vi "Run Filter.vi"(8 "error in (no error)":errorcluster, 10 "fpga resources in":T1[](array[typedef]), 11 "OR Filter in":refnum<class "OR Filter.lvclass">) -> (0 "error out":errorcluster, 2 "fpga resources in":T1[](array[typedef]))   [LabVIEW 2016, in "OR Filter.lvclass"]
uses:
  OR Filter.lvclass
  FPGA-Addon/Source/System Explorer/SubVIs/fpga resource.ctl
  FPGA-Addon/Source/System Explorer/SubVIs/Channel Type.ctl
  OR Filter.lvclass/OR Filter.ctl
  Filter Parent/Filter.lvclass
  FPGA-Addon/Source/System Explorer/FPGA Addon System Explorer.lvlib
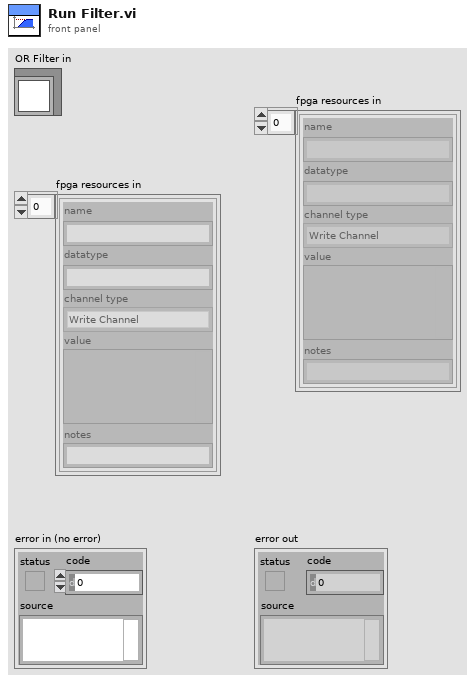
[diagram p1: front panel]
types:
  T1 = typedef "FPGA Addon System Explorer.lvlib/fpga resource.ctl" = cluster{"name":string, "datatype":string, "channel type":T2, "value":variant, "notes":string}
  T2 = typedef "FPGA Addon System Explorer.lvlib/Channel Type.ctl" = enum16{"Write Channel", "Read Channel", "Write Waveform", "Read Waveform"}
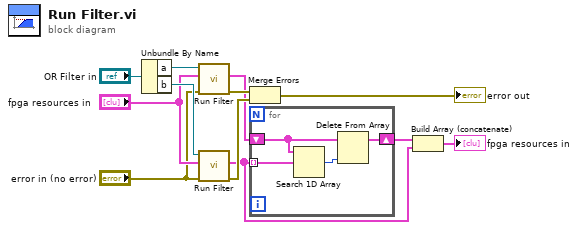
[diagram p0: block diagram]
diagram:
  n1 = Unbundle By Name("OR Filter in") -> ("a"=w11:refnum<class "Filter.lvclass">, "b"=w10:refnum<class "Filter.lvclass">)
  n2 = call-dynamic "Run Filter.vi"("error in (no error)"="error in (no error)", "fpga resources in"="fpga resources in", "Filter in"=w11) -> ("error out"=w7:errorcluster, "fpga resources out"=w4:T1[])  [unwired: 7 in]
  n3 = call-dynamic "Run Filter.vi"("error in (no error)"="error in (no error)", "fpga resources in"="fpga resources in", "Filter in"=w10) -> ("error out"=w6:errorcluster, "fpga resources out"=w2:T1[])  [unwired: 7 in]
  n4 = Merge Errors(w7, w6) -> (→"error out":errorcluster)
  n5 = for {
    tunnel: w2 -> [w16] mode=indexing
    shift-right: [w13] -> w3
    shift-left: w4 -> [w14]
    n6 = Search 1D Array(1D array=w14, element=w16) -> (index of element=w15:i32)  [unwired: 1 in]
    n7 = Delete From Array(array=w14, index=w15) -> (array with subset deleted=w13:T1[])  [unwired: 1 in, 1 out]
  }
  n8 = Build Array (concatenate)(w3, w2) -> (→"fpga resources in":T1[])
